vi "MessageCorrect.vi"(1 "Test":i8[](array[numeric]), 2 "Sample":u8[](array[numeric])) -> (0 "BER":dbl)   [LabVIEW 2014]
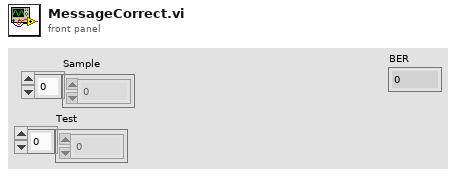
[diagram p1: front panel]
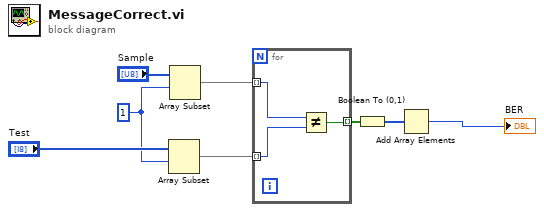
[diagram p0: block diagram]
diagram:
  w3 = 1
  n1 = Array Subset(array="Test", index=w3) -> (w4:i8[])  [unwired: 1 in]
  n2 = Array Subset(array="Sample", index=w3) -> (w2:u8[])  [unwired: 1 in]
  n3 = for {
    tunnel: w2 -> [w11] mode=indexing
    tunnel: w4 -> [w10] mode=indexing
    tunnel: [w9] -> w8 mode=indexing
    n4 = Not Equal?(x=w11, y=w10) -> (x != y?=w9:bool)
  }
  n5 = Boolean To (0,1)(Boolean=w8) -> (0, 1=w7:i16[])
  n6 = Add Array Elements(numeric array=w7) -> (sum=→"BER":i16)
